vi "Exp_SetExposuresPerFrame.vi"(8 "error in (no error)":errorcluster, 10 "Exposures Per Frame":i32, 11 "LightField Automation in":refnum<class "LightField Automation.lvclass">) -> (0 "error out":errorcluster, 3 "LightField Automation out":refnum<class "LightField Automation.lvclass">)   [LabVIEW 2013, in "LightField Automation.lvclass"]
uses:
  LightField Automation.lvclass
  LightField Automation.lvclass/LightField Automation.ctl
  C:/Program Files/Princeton Instruments/LightField/PrincetonInstruments.LightFieldAddInSupportServices.dll
  Program Files/Princeton Instruments/LightField/PrincetonInstruments.LightFieldAddInSupportServices.dll
  C:/Program Files/Princeton Instruments/LightField/AddInViews/PrincetonInstruments.LightFieldViewV3.dll
  Program Files/Princeton Instruments/LightField/AddInViews/PrincetonInstruments.LightFieldViewV3.dll
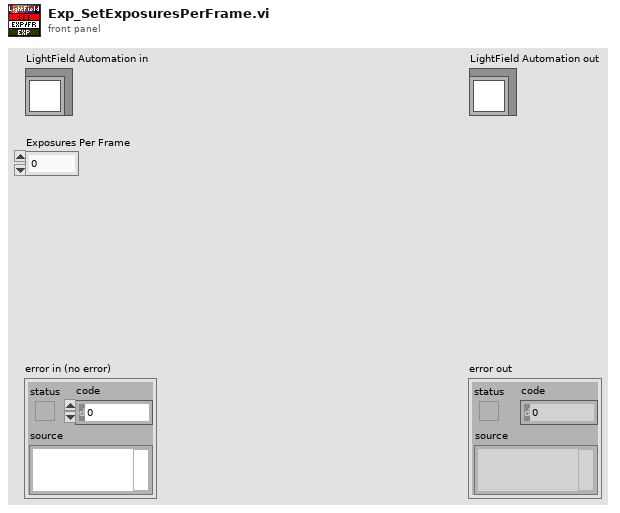
[diagram p1: front panel]
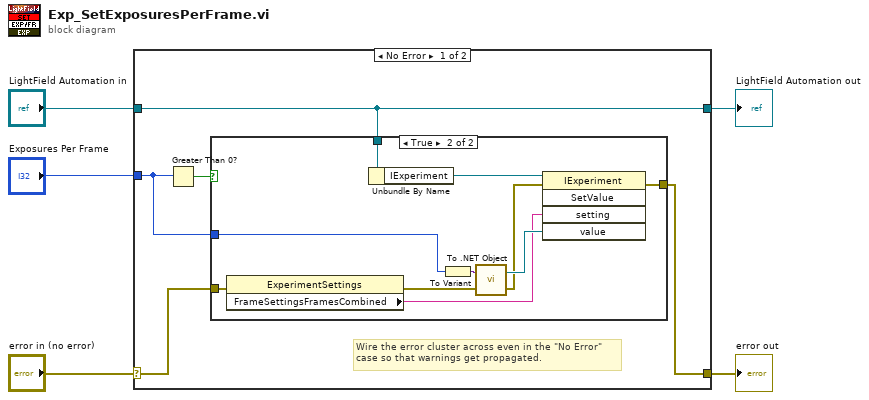
[diagram p0: block diagram]
diagram:
  n1 = case shown="No Error" "error in (no error)" {
    selector: "error in (no error)" -> [w8 w23]
    tunnel: [w6 w23] -> w4
    tunnel: [w7 w22] -> w2
    tunnel: "LightField Automation in" -> [w7 w22]
    tunnel: "Exposures Per Frame" -> [w9 _]
    frame No Error {
      # "Wire the error cluster across even in the \"No Error\"\ncase so that warnings get propagated."
      n2 = Greater Than 0?(x=w9) -> (x > 0?=w10:bool)
      n3 = case shown="True" w10 {
        tunnel: w9 -> [_ w21]
        tunnel: w8 -> [w11 w14]
        tunnel: w7 -> [_ w17]
        tunnel: [w11 w15] -> w6
        frame False {
        }
        frame True {
          n4 = property class="ExperimentSettings"(error in=w14) -> (error out=w12:errorcluster, "FrameSettingsFramesCombined"=w13:string)  [unwired: 1 in, 1 out]
          n5 = Unbundle By Name(w17) -> ("IExperiment"=w16:refnum<k24>)
          n6 = To Variant(anything=w21) -> (Variant=w20:variant)
          n7 = call <vilib>:"To .NET Object.vi"("error in (no error)"=w12, "anything"=w20) -> ("error out"=w18:errorcluster, ".NET object"=w19:refnum<k24>)
          n8 = invoke class="IExperiment" method="SetValue"(reference=w16, error in=w18, "setting"=w13, "value"=w19) -> (error out=w15:errorcluster)  [unwired: 1 in, 4 out]
        }
      }
    }
    frame Error {
    }
  }
  "error out" <- w4
  "LightField Automation out" <- w2
